vi "Read Ignore Attributes.vi"(8 "error in (no error)":errorcluster, 11 "WaveformGraph.lvclass in":refnum<class "WaveformGraph.lvclass">) -> (0 "error out":errorcluster, 2 "IgnoreAttributes":bool, 3 "WaveformGraph.lvclass out":refnum<class "WaveformGraph.lvclass">)   [LabVIEW 2015, in "WaveformGraph.lvclass"]
uses:
  WaveformGraph.lvclass
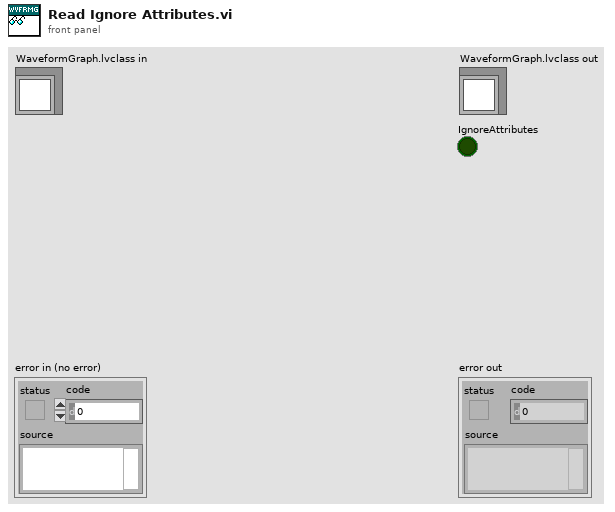
[diagram p1: front panel]
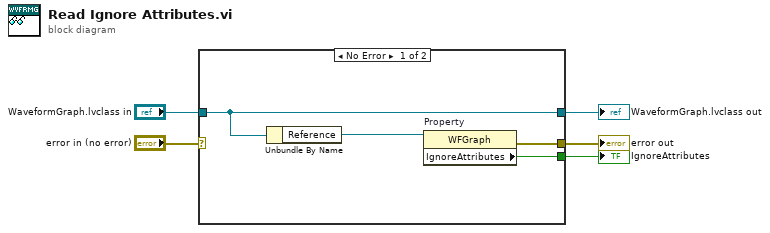
[diagram p0: block diagram]
diagram:
  n1 = case shown="No Error" "error in (no error)" {
    selector: "error in (no error)" -> [_ w11]
    tunnel: [w8 w11] -> w4
    tunnel: [w7 w10] -> w2
    tunnel: "WaveformGraph.lvclass in" -> [w7 w10]
    tunnel: [w9 _] -> w1
    frame No Error {
      n2 = Unbundle By Name(w7) -> ("Reference"=w6:refnum<vi>)
      n3 = property on="Property" class="WFGraph"(reference=w6) -> (error out=w8:errorcluster, "IgnoreAttributes"=w9:bool)  [unwired: 1 in, 1 out]
    }
    frame Error {
    }
  }
  "error out" <- w4
  "WaveformGraph.lvclass out" <- w2
  "IgnoreAttributes" <- w1
